vi "Gate Defense.vi"(10 "Arm Function":enum16{"Up", "Down"}(ring)) -> ()   [LabVIEW 2015]
uses:
  Robot Global.vi
  <vilib>/Rock Robotics/WPI/CAN/Jaguar/SubVIs/WPI_CANJaguar_ControlMode.ctl
  <vilib>/Rock Robotics/WPI/CAN/TalonSRX/WPI_CANTalonSRX_APIControlMode.ctl
  <vilib>/Rock Robotics/SystemInterfaces/DIO/FPGA_DIOPWMChannel.ctl
  <vilib>/Rock Robotics/WPI/PWM/WPI_PWMDeadband.ctl
  <vilib>/Rock Robotics/WPI/MotorControl/WPI_MotorControlType.ctl
  <vilib>/Rock Robotics/WPI/MotorControl/WPI_MotorControlDeviceRef.ctl
  <vilib>/Rock Robotics/SystemInterfaces/DIO/FPGA_DIOChannel.ctl
  <vilib>/Rock Robotics/WPI/DigitalInput/WPI_DigitalInputDevRef.ctl
panel:
  out "Right Arm Sensor":T1
  out "Left Arm Sensor":T1
  out "Right Arm Motor":T3={"DeviceStatus"={"status"=FALSE, "code"=0, "source"=""}, "Type"=enum."PWM", "PWM"={"PWM Channel"=enum."Invalid", "DeadBand"={"Name"="", "maxPositivePwm"=0, "minPositivePwm"=0, "centerPwm"=0, "maxNegativePwm"=0, "minNegativePwm"=0, "angularRange"=0}}, "CAN"={"Device Number"=0, "Control Mode"=enum."Percent VBus", "Semaphore"=refnum, "Max Vout"=12.0, "TalonSRX Control Mode"=enum."Percent VBus"}, "Invert"=FALSE}
  out "Left Arm Motor":T3={"DeviceStatus"={"status"=FALSE, "code"=0, "source"=""}, "Type"=enum."PWM", "PWM"={"PWM Channel"=enum."Invalid", "DeadBand"={"Name"="", "maxPositivePwm"=0, "minPositivePwm"=0, "centerPwm"=0, "maxNegativePwm"=0, "minNegativePwm"=0, "angularRange"=0}}, "CAN"={"Device Number"=0, "Control Mode"=enum."Percent VBus", "Semaphore"=refnum, "Max Vout"=12.0, "TalonSRX Control Mode"=enum."Percent VBus"}, "Invert"=FALSE}
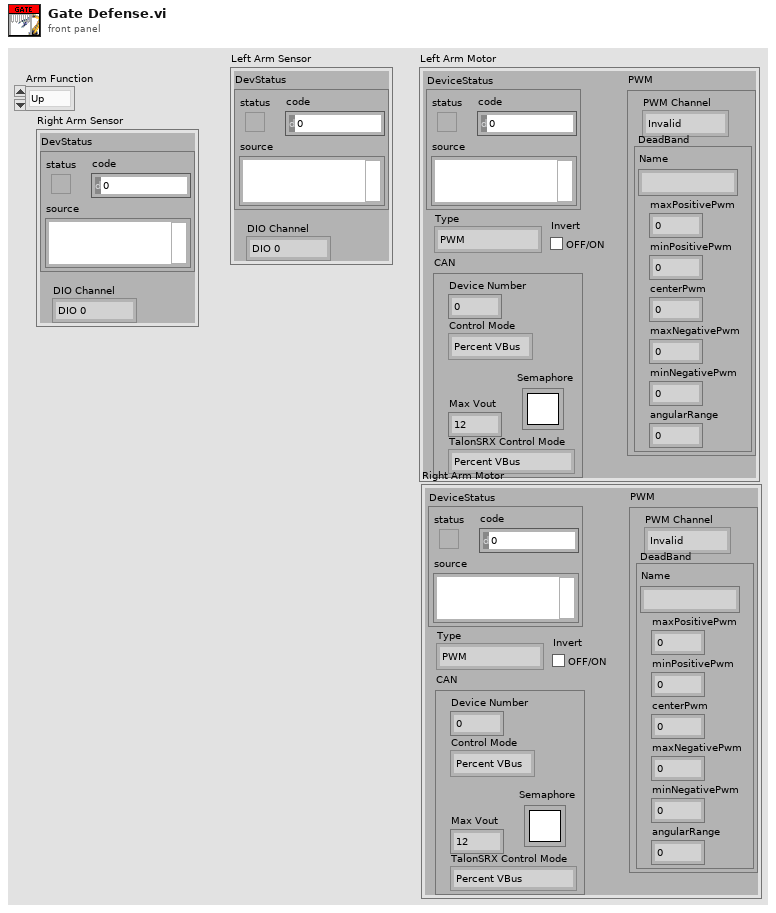
[diagram p1: front panel]
types:
  T1 = typedef "WPI_DigitalInputDevRef.ctl" = cluster{"DevStatus":errorcluster, "DIO Channel":T2}
  T2 = typedef "FPGA_DIOChannel.ctl" = enum8{"DIO 0", "DIO 1", "DIO 2", "DIO 3", "DIO 4", "DIO 5", "DIO 6", "DIO 7", "DIO 8", "DIO 9", "DIO MXP 0", "DIO MXP 1", "DIO MXP 2", "DIO MXP 3", "DIO MXP 4", "DIO MXP 5", "DIO MXP 6", "DIO MXP 7", "DIO MXP 8", "DIO MXP 9", "DIO MXP 10", "DIO MXP 11", "DIO MXP 12", "DIO MXP 13", "DIO MXP 14", "DIO MXP 15", "Invalid"}
  T3 = typedef "WPI_MotorControlDeviceRef.ctl" = cluster{"DeviceStatus":errorcluster, "Type":T4, "PWM":cluster{"PWM Channel":T5, "DeadBand":T6}, "CAN":cluster{"Device Number":u8, "Control Mode":T7, "Semaphore":T8, "Max Vout":dbl, "TalonSRX Control Mode":T9}, "Invert":bool}
  T4 = typedef "WPI_MotorControlType.ctl" = enum16{"PWM", "CAN", "CANTalonSRX"}
  T5 = typedef "FPGA_DIOPWMChannel.ctl" = enum8{"PWM 0", "PWM 1", "PWM 2", "PWM 3", "PWM 4", "PWM 5", "PWM 6", "PWM 7", "PWM 8", "PWM 9", "PWM MXP 0", "PWM MXP 1", "PWM MXP 2", "PWM MXP 3", "PWM MXP 4", "PWM MXP 5", "PWM MXP 6", "PWM MXP 7", "PWM MXP 8", "PWM MXP 9", "Invalid"}
  T6 = typedef "WPI_PWMDeadband.ctl" = cluster{"Name":string, "maxPositivePwm":i32, "minPositivePwm":i32, "centerPwm":i32, "maxNegativePwm":i32, "minNegativePwm":i32, "angularRange":u16}
  T7 = typedef "WPI_CANJaguar_ControlMode.ctl" = enum8{"Percent VBus", "Current", "Speed", "Position", "Voltage"}
  T8 = typedef "Semaphore RefNum" = refnum<k1>
  T9 = typedef "WPI_CANTalonSRX_APIControlMode.ctl" = enum8{"Percent VBus", "Speed", "Position", "Slave", "Unchanged / Invalid", "Voltage Compensation", "Current", "Motion Profile"}
  T10 = typedef "Robot Drive.ctl" = cluster{"RobotDriveDevRef":T11, "Joysticks":cluster{"JoystickDevRef":T12, "JoystickDevRef 2":T12}, "Sensor":cluster{"GyroDevRef":T14, "Left Arm DigitalInputDevRef":T1, "Right ArmDigitalInputDevRef":T1, "Hanging DigitalInputDevRef":T1, "Left Arm EncoderDevRef":T17, "Right Arm EncoderDevRef":T17, "Left Drive EncoderDevRef":T17, "Right Drive EncoderDevRef":T17, "BoB SonarMB1010AnalogDevRef":T21}, "Aquisition + Scoring":cluster{"Aquisition MotorControlDeviceRef":T3, "Scoring 1 MotorControlDeviceRef":T3, "Scoring 2 MotorControlDeviceRef":T3}, "Pneumatics":cluster{"CompressorDevRef":T23, "High and Low Gear DoubleSolenoidDevRef":T24, "PTO SignleSolenoidDevRef":T24, "Shooter SolenoidDevRef":T24, "Drive Neutral SolenoidDevRef":T24}, "Defenses":cluster{"LeftArm MotorControlDeviceRef":T3, "RightArm MotorControlDeviceRef":T3, "Roller MotorControlDeviceRef":T3}, "Hanging":cluster{"Erection MotorControlDeviceRef":T3}}
  T11 = typedef "WPI_RobotDriveDevRef.ctl" = cluster{"DevStatus":errorcluster, "Motors[]":T3[], "Square Inputs":bool, "Max Output":dbl}
  T12 = typedef "WPI_JoystickDevRef.ctl" = cluster{"Device":T13}
  T13 = typedef "WPI_JoystickDeviceEnum.ctl" = enum16{"USB 0", "USB 1", "USB 2", "USB 3", "USB 4", "USB 5"}
  T14 = typedef "WPI_GyroDevRef.ctl" = cluster{"DevStatus":errorcluster, "Analog Channel":T15, "Offset":dbl, "Gain (VoltsPerDegree/Second)":dbl, "Gyro Type":enum16{"Analog", "XRS450"}, "Handle":i32, "SPI Bus":T16, "Device Found":bool, "Sample Rate":dbl, "Calibrate On Open":bool}
  T15 = typedef "FPGA_AIChannel.ctl" = enum8{"AI 0", "AI 1", "AI 2", "AI 3", "AI MXP 0", "AI MXP 1", "AI MXP 2", "AI MXP 3", "Invalid"}
  T16 = typedef "spi_bus.ctl" = enum16{"SPI On-Board, CS0", "SPI On-Board, CS1", "SPI On-Board, CS2", "SPI On-Board, CS3", "SPI MXP", "Invalid"}
  T17 = typedef "WPI_EncoderDevRef.ctl" = cluster{"DevStatus":errorcluster, "EncoderIndex":T18, "CounterIndex":T19, "DistancePerCount":dbl, "Decoding Type":T20}
  T18 = typedef "FPGA_EncoderIdx.ctl" = enum8{"Enc 0", "Enc 1", "Enc 2", "Enc 3", "Enc 4", "Enc 5", "Enc 6", "Enc 7", "Invalid"}
  T19 = typedef "FPGA_CounterCtrSystemIndex.ctl" = enum8{"Ctr 0", "Ctr 1", "Ctr 2", "Ctr 3", "Ctr 4", "Ctr 5", "Ctr 6", "Ctr 7", "Invalid"}
  T20 = typedef "WPI_EncoderType.ctl" = enum16{"1x", "2x", "4x"}
  T21 = typedef "WPI_SonarMB1010AnalogDeviceRef.ctl" = cluster{"AIDeviceRef":T22, "Scaling factor (V/in)":dbl, "Average Bits":u8}
  T22 = typedef "WPI_AnalogChannelDevRef.ctl" = cluster{"DevStatus":errorcluster, "Analog Channel":T15}
  T23 = typedef "WPI_CompressorDevRef.ctl" = cluster{"DevStatus":errorcluster, "Pneumatics Control Module":u8}
  T24 = typedef "WPI_SolenoidDevRef.ctl" = cluster{"DevStatus":errorcluster, "Pneumatics Control Module":u8, "Forward Solenoid Channel":T25, "Reverse Solenoid Channel":T25}
  T25 = typedef "WPI_SolenoidChannel.ctl" = enum8{"Solenoid 0", "Solenoid 1", "Solenoid 2", "Solenoid 3", "Solenoid 4", "Solenoid 5", "Solenoid 6", "Solenoid 7", "Invalid"}
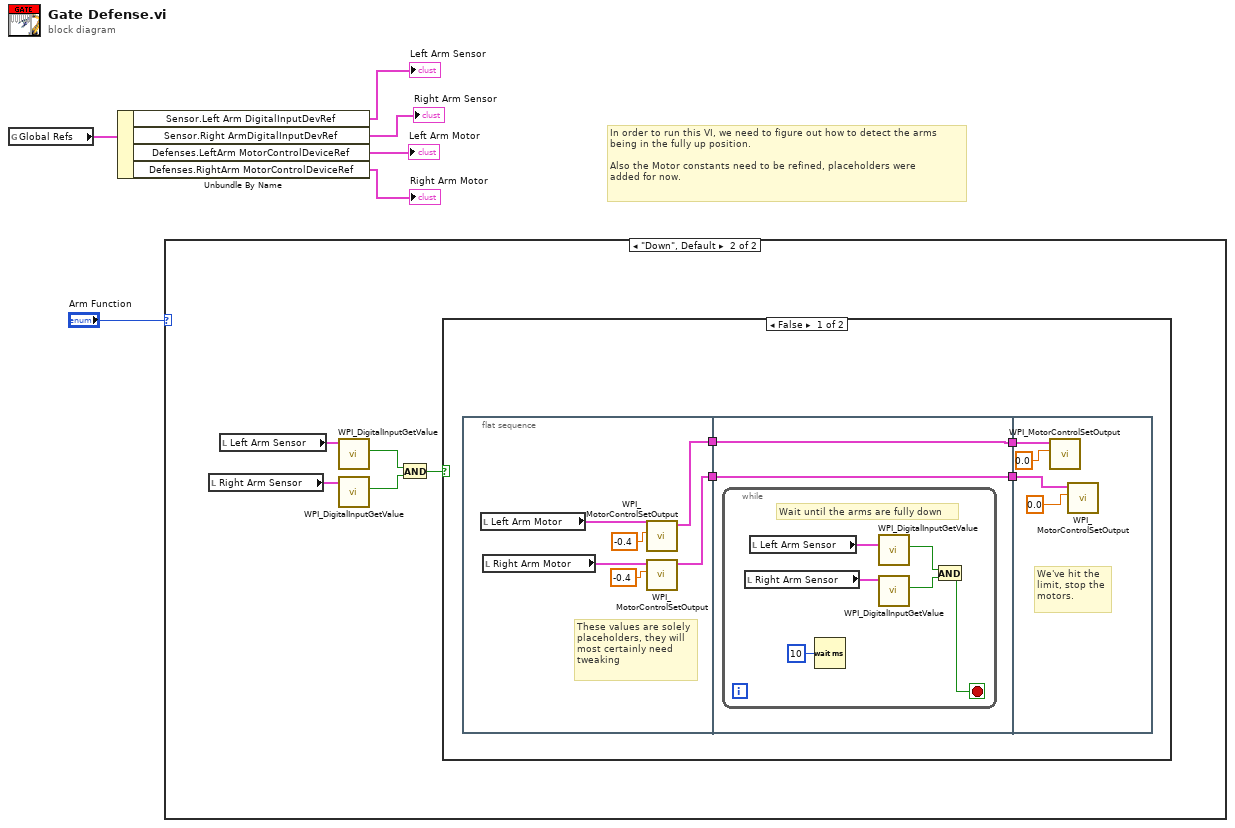
[diagram p0: block diagram]
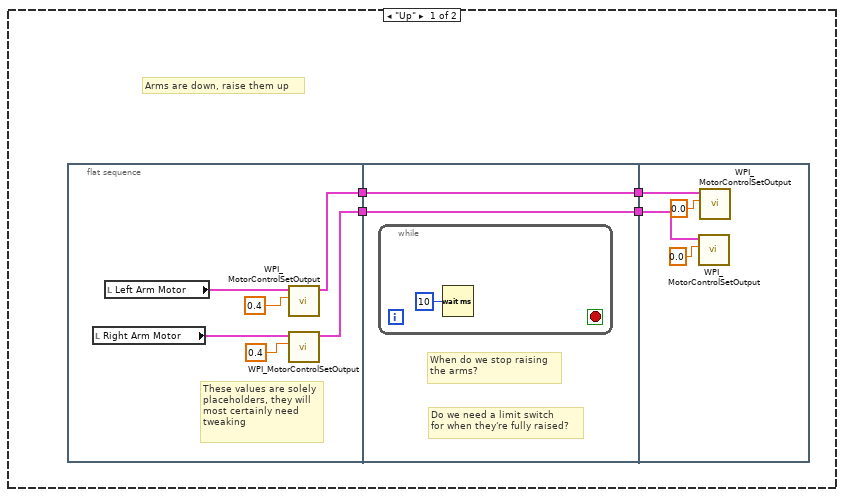
[diagram p2: hidden frame]
diagram:
  # "In order to run this VI, we need to figure out how to detect the arms\nbeing in the fully up position.\n\nAlso the Motor constants need to be refined, placeholders were\nadded for now."
  n1 = global read "Robot Global.vi" "Global Refs"() -> (w6:T10)
  n2 = Unbundle By Name(w6) -> ("Sensor.Left Arm DigitalInputDevRef"=→"Left Arm Sensor":T1, "Sensor.Right ArmDigitalInputDevRef"=→"Right Arm Sensor":T1, "Defenses.LeftArm MotorControlDeviceRef"=→"Left Arm Motor":T3, "Defenses.RightArm MotorControlDeviceRef"=→"Right Arm Motor":T3)
  n3 = case shown="\"Down\", Default" "Arm Function" {
    frame "Up" {
      # "Arms are down, raise them up"
      n4 = flat-sequence {
        tunnel: [w12] -> w10
        tunnel: [w11] -> w7
        tunnel: w10 -> [w18]
        tunnel: [w18] -> w9
        tunnel: [w17] -> w8
        tunnel: w7 -> [w17]
        tunnel: w9 -> [w21]
        tunnel: w8 -> [w20]
        frame #0 {
          # "These values are solely\nplaceholders, they will\nmost certainly need\ntweaking"
          n5 = local read "Right Arm Motor"() -> (w13:T3)
          n6 = local read "Left Arm Motor"() -> (w14:T3)
          n7 = call <vilib>:"WPI_MotorControlSetOutput.vi"("Output"=0.4, "MotorControlDevRef"=w14) -> ("MotorControlDevRef"=w12:T3)  [unwired: 7 in, 2 out]
          n8 = call <vilib>:"WPI_MotorControlSetOutput.vi"("Output"=0.4, "MotorControlDevRef"=w13) -> ("MotorControlDevRef"=w11:T3)  [unwired: 7 in, 2 out]
        }
        frame #1 {
          # "When do we stop raising\nthe arms?"
          # "Do we need a limit switch\nfor when they're fully raised?"
          n9 = while {
            stop <- _ stop-if-true
            n10 = Wait (ms)(milliseconds to wait=u32 10) -> ()  [unwired: 1 out]
          }
        }
        frame #2 {
          n11 = call <vilib>:"WPI_MotorControlSetOutput.vi"("Output"=0.0, "MotorControlDevRef"=w20) -> ()  [unwired: 7 in, 3 out]
          n12 = call <vilib>:"WPI_MotorControlSetOutput.vi"("Output"=0.0, "MotorControlDevRef"=w21) -> ()  [unwired: 7 in, 3 out]
        }
      }
    }
    frame "Down", Default {
      n13 = local read "Right Arm Sensor"() -> (w24:T1)
      n14 = local read "Left Arm Sensor"() -> (w25:T1)
      n15 = call <vilib>:"WPI_DigitalInputGetValue.vi"("DigitalInputDevRef"=w25) -> ("Value"=w28:bool)  [unwired: 8 in, 2 out]
      n16 = call <vilib>:"WPI_DigitalInputGetValue.vi"("DigitalInputDevRef"=w24) -> ("Value"=w27:bool)  [unwired: 8 in, 2 out]
      n17 = And(x=w28, y=w27) -> (x .and. y?=w26:bool)
      n18 = case shown="False" w26 {
        frame False {
          n19 = flat-sequence {
            tunnel: [w34] -> w31
            tunnel: [w33] -> w30
            tunnel: [w40] -> w32
            tunnel: w31 -> [w40]
            tunnel: w30 -> [w39]
            tunnel: [w39] -> w29
            tunnel: w32 -> [w50]
            tunnel: w29 -> [w47]
            frame #0 {
              # "These values are solely\nplaceholders, they will\nmost certainly need\ntweaking"
              n20 = local read "Left Arm Motor"() -> (w36:T3)
              n21 = local read "Right Arm Motor"() -> (w35:T3)
              n22 = call <vilib>:"WPI_MotorControlSetOutput.vi"("Output"=-0.4, "MotorControlDevRef"=w36) -> ("MotorControlDevRef"=w34:T3)  [unwired: 7 in, 2 out]
              n23 = call <vilib>:"WPI_MotorControlSetOutput.vi"("Output"=-0.4, "MotorControlDevRef"=w35) -> ("MotorControlDevRef"=w33:T3)  [unwired: 7 in, 2 out]
            }
            frame #1 {
              n24 = while {
                stop <- w44 stop-if-true
                # "Wait until the arms are fully down"
                n25 = local read "Right Arm Sensor"() -> (w41:T1)
                n26 = local read "Left Arm Sensor"() -> (w42:T1)
                n27 = Wait (ms)(milliseconds to wait=u32 10) -> ()  [unwired: 1 out]
                n28 = call <vilib>:"WPI_DigitalInputGetValue.vi"("DigitalInputDevRef"=w42) -> ("Value"=w46:bool)  [unwired: 8 in, 2 out]
                n29 = call <vilib>:"WPI_DigitalInputGetValue.vi"("DigitalInputDevRef"=w41) -> ("Value"=w45:bool)  [unwired: 8 in, 2 out]
                n30 = And(x=w46, y=w45) -> (x .and. y?=w44:bool)
              }
            }
            frame #2 {
              # "We've hit the\nlimit, stop the\nmotors."
              n31 = call <vilib>:"WPI_MotorControlSetOutput.vi"("Output"=0.0, "MotorControlDevRef"=w50) -> ()  [unwired: 7 in, 3 out]
              n32 = call <vilib>:"WPI_MotorControlSetOutput.vi"("Output"=0.0, "MotorControlDevRef"=w47) -> ()  [unwired: 7 in, 3 out]
            }
          }
        }
        frame True {
          # "The arms are already down!"
        }
      }
    }
  }
